vi "set_PulseWidthAUX2.vi"() -> ()   [LabVIEW 2014]
panel:
  in  "Address (0x50)":u16=80 max=1023 format="%.0x"
  in  "Aardvark Handle":i32 min=0
  out "error out":errorcluster
  in  "error in (no error)":errorcluster
  in  "Pulsewidth":dbl
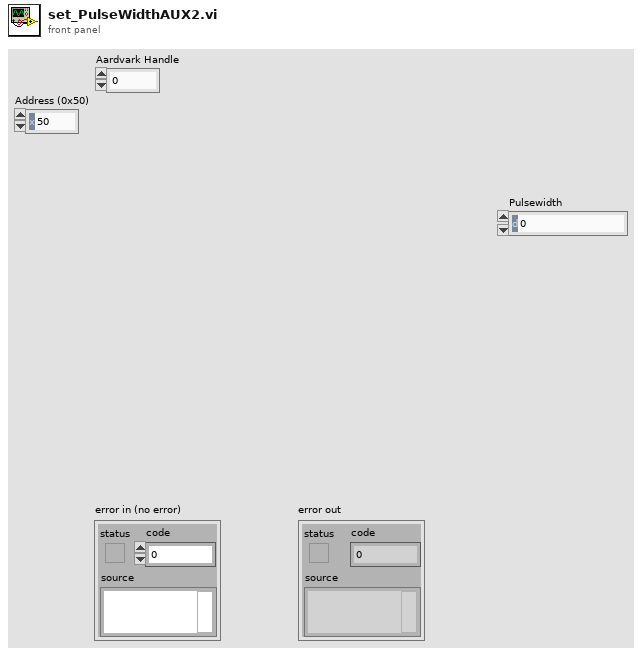
[diagram p1: front panel]
types:
  T1 = cluster{"unsigned byte array[0]":u8, "unsigned byte array[1]":u8, "unsigned byte array[2]":u8, "unsigned byte array[3]":u8, "unsigned byte array[4]":u8, "unsigned byte array[5]":u8, "unsigned byte array[6]":u8, "unsigned byte array[7]":u8, "unsigned byte array[8]":u8}
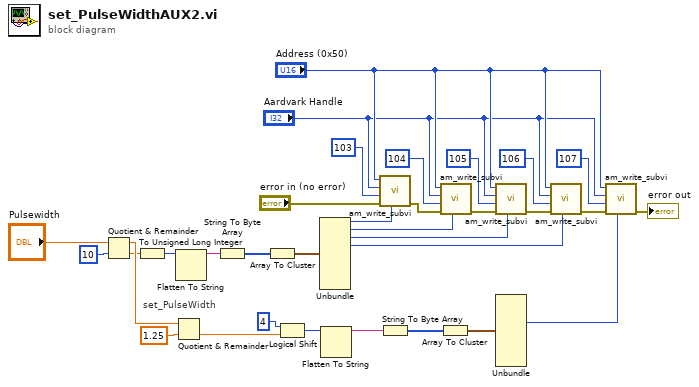
[diagram p0: block diagram]
diagram:
  # "set_PulseWidth"
  n1 = Quotient & Remainder(x="Pulsewidth", y=10) -> (x-y*floor(x/y)=w31:dbl, floor(x/y)=w24:dbl)
  n2 = To Unsigned Long Integer(number=w24) -> (unsigned 32bit integer=w23:u32)
  n3 = Quotient & Remainder(x=w31, y=1.25) -> (floor(x/y)=w28:dbl)  [unwired: 1 out]
  n4 = Flatten To String(anything=w23) -> (data string=w27:string)  [unwired: 3 in, 2 out]
  n5 = String To Byte Array(string=w27) -> (unsigned byte array=w22:u8[])
  n6 = Array To Cluster(array=w22) -> (cluster=w21:T1)
  n7 = Logical Shift(y=4, x=w28) -> (x << y=w25:u32)
  n8 = Unbundle(w21) -> ("unsigned byte array[0]"=w5:u8, "unsigned byte array[1]"=w4:u8, "unsigned byte array[2]"=w3:u8, "unsigned byte array[3]"=w2:u8)  [unwired: 5 out]
  n9 = Flatten To String(anything=w25) -> (data string=w26:string)  [unwired: 3 in, 2 out]
  n10 = call "am_write_subvi.vi"("Data to Write"=w5, "error in (no error)"="error in (no error)", "Memory ADD"=u16 103, "Aardvark Handle in"="Aardvark Handle", "Address (0x50) in"="Address (0x50)") -> ("error out"=w17:errorcluster)  [unwired: 5 in, 1 out]
  n11 = String To Byte Array(string=w26) -> (unsigned byte array=w20:u8[])
  n12 = Array To Cluster(array=w20) -> (cluster=w19:T1)
  n13 = call "am_write_subvi.vi"("Data to Write"=w4, "error in (no error)"=w17, "Memory ADD"=u16 104, "Aardvark Handle in"="Aardvark Handle", "Address (0x50) in"="Address (0x50)") -> ("error out"=w16:errorcluster)  [unwired: 5 in, 1 out]
  n14 = call "am_write_subvi.vi"("Data to Write"=w3, "error in (no error)"=w16, "Memory ADD"=u16 105, "Aardvark Handle in"="Aardvark Handle", "Address (0x50) in"="Address (0x50)") -> ("error out"=w15:errorcluster)  [unwired: 5 in, 1 out]
  n15 = Unbundle(w19) -> ("unsigned byte array[3]"=w1:u8)  [unwired: 8 out]
  n16 = call "am_write_subvi.vi"("Data to Write"=w2, "error in (no error)"=w15, "Memory ADD"=u16 106, "Aardvark Handle in"="Aardvark Handle", "Address (0x50) in"="Address (0x50)") -> ("error out"=w14:errorcluster)  [unwired: 5 in, 1 out]
  n17 = call "am_write_subvi.vi"("Data to Write"=w1, "error in (no error)"=w14, "Memory ADD"=u16 107, "Aardvark Handle in"="Aardvark Handle", "Address (0x50) in"="Address (0x50)") -> ("error out"=→"error out":errorcluster)  [unwired: 5 in, 1 out]
